vi "Sub_get_eigensol_and_sort_native_LABView.vi"(0 "Mass":T1, 1 "Stiffness":T1) -> (14 "Unsorted Eigenvalues":dbl[](array[numeric]), 15 "Sorted Eigenvalues":dbl[](array[numeric]), 16 "Unsorted Eigenvector Matrix":T1, 17 "Sorted Eigenvector Matrix":T1, 18 "Natural frequency":dbl[](array[numeric]))   [LabVIEW 2021]
uses:
  <vilib>/Analysis/Matrix/Datatypes/RealMatrix.ctl
  <vilib>/Analysis/Matrix/Numeric/Conversions/Matrix To Array - RM.vi
  <vilib>/Analysis/Matrix/Numeric/Conversions/Array To Matrix - RA2.vi
  <vilib>/Analysis/Matrix/NI_Matrix.lvlib
panel:
  # "Inputs"
  # "Outputs"
  # "This is a wrapper for Sub_Python_cmd_eigh.vi that sorts the eigen values returns the values of intrerest, IF YOU REPLACE the sub_vi this VI will sort the eigenvectors by ascending order according to their corresponding eigenvalues ASUMMING that the eigenvalues are stored as a vector V[i] corresonds to each column in eigenvector matrix W[:,i ]. Not all eigensolvers sort their eigenvalues in a simple ascending or descending order, or any order for that matter. This VI performs simple sort naive to any presupposed ordering.\n\n              - Alexander Vereen AFRL Summer scholars 2022"
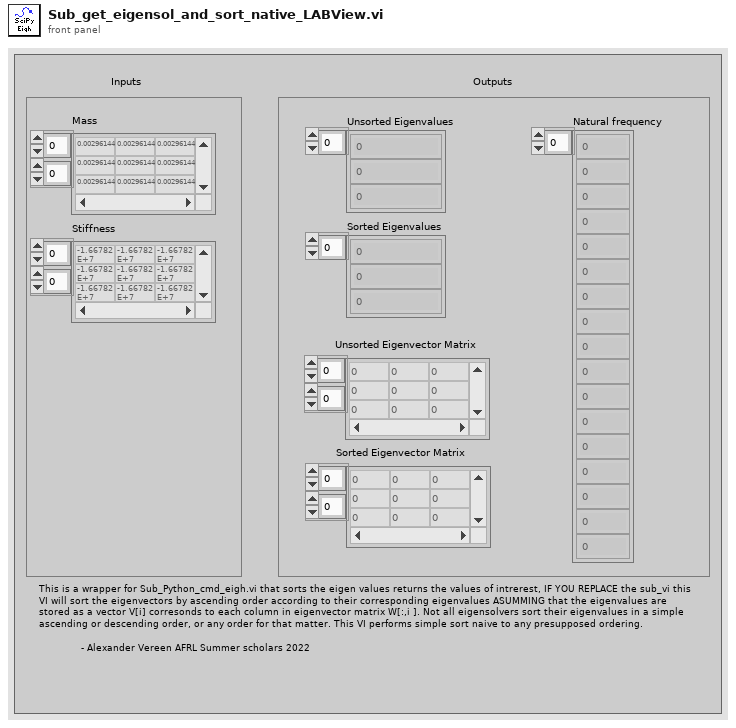
[diagram p1: front panel]
types:
  T1 = typedef "NI_Matrix.lvlib/RealMatrix.ctl" = dbl[][]
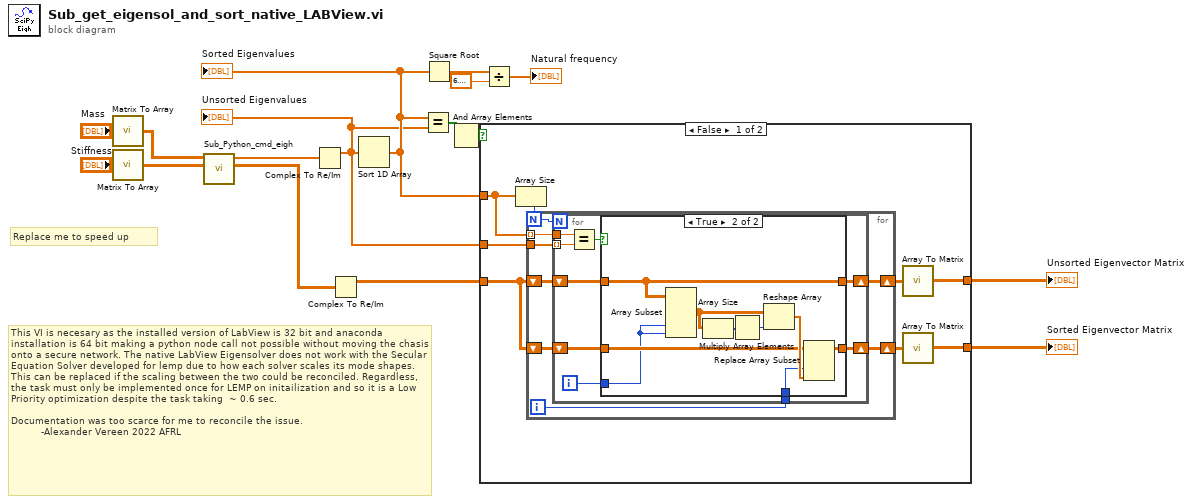
[diagram p0: block diagram]
diagram:
  # "Replace me to speed up"
  # "This VI is necesary as the installed version of LabView is 32 bit and anaconda installation is 64 bit making a python node call not possible without moving the chasis onto a secure network. The native LabView Eigensolver does not work with the Secular Equation Solver developed for lemp due to how each solver scales its mode shapes.  This can be replaced if the scaling between the two could be reconciled. Regardless, the task must only be implemented once for LEMP on initailization and so it is a Low Priority optimization despite the task taking  ~ 0.6 sec. \n\nDocumentation was too scarce for me to reconcile the issue.\n          -Alexander Vereen 2022 AFRL"
  n1 = call-poly <vilib>:"Matrix To Array.vi"("Real Matrix"="Mass") -> ("Real 2D Array"=w5:dbl[][])
  n2 = call-poly <vilib>:"Matrix To Array.vi"("Real Matrix"="Stiffness") -> ("Real 2D Array"=w6:dbl[][])
  n3 = call "Sub_Python_cmd_eigh.vi"("Stiff"=w6, "Mass"=w5) -> ("Eigenvectors"=w8:dbl[][], "Eigenvalues"=w9:dbl[])  [unwired: 8 in]
  n4 = Complex To Re/Im ("Complex To Cartesian.vi")(x + iy=w9) -> (x=w3:dbl[])  [unwired: 1 out]
  "Unsorted Eigenvalues" <- w3
  n5 = Complex To Re/Im ("Complex To Cartesian.vi")(x + iy=w8) -> (x=w12:dbl[][])  [unwired: 1 out]
  n6 = Sort 1D Array(array=w3) -> (sorted array=w4:dbl[])
  "Sorted Eigenvalues" <- w4
  n7 = Equal?(x=w4, y=w3) -> (x = y?=w2:bool[])
  n8 = Square Root ("Square Root.vi")(x=w4) -> (sqrt(x)=w16:dbl[])
  n9 = And Array Elements(Boolean array=w2) -> (logical AND=w1:bool)
  n10 = case shown="False" w1 {
    tunnel: [w21 w53] -> w14
    tunnel: [w20 w53] -> w13
    tunnel: w12 -> [w19 w53]
    tunnel: w3 -> [w18 _]
    tunnel: w4 -> [w17 _]
    frame False {
      n11 = Array Size(array=w17) -> (size(s)=w24:i32)
      n12 = for {
        N: w24 -> [w25]
        tunnel: w17 -> [w31] mode=indexing
        tunnel: w18 -> [w32]
        shift-right: [w29] -> w23
        shift-left: w19 -> [w30]
        shift-right: [w27] -> w22
        shift-left: w19 -> [w26]
        i -> [w28]
        n13 = for {
          N: w25 -> [_]
          tunnel: w32 -> [w40] mode=indexing
          tunnel: w31 -> [w41]
          shift-right: [w37] -> w29
          shift-left: w30 -> [w38]
          tunnel: w28 -> [w36]
          shift-right: [w34] -> w27
          shift-left: w26 -> [w33]
          i -> [w35]
          n14 = Equal?(x=w41, y=w40) -> (x = y?=w39:bool)
          n15 = case shown="True" w39 {
            tunnel: w38 -> [w43 w47]
            tunnel: [w43 w47] -> w37
            tunnel: w36 -> [_ w46]
            tunnel: w35 -> [_ w45]
            tunnel: [w42 w49] -> w34
            tunnel: w33 -> [w42 w48]
            frame False {
            }
            frame True {
              n16 = Array Subset(array=w47, index (col)=w45, length (col)=w45) -> (w50:dbl[][])  [unwired: 2 in]
              n17 = Array Size(array=w50) -> (size(s)=w51:i32[])
              n18 = Multiply Array Elements(1:w51) -> (0:w44:i32)
              n19 = Reshape Array(w50, w44) -> (w52:dbl[])
              n20 = Replace Array Subset(array=w48, new element=w52, index (col)=w46) -> (w49:dbl[][])  [unwired: 1 in]
            }
          }
        }
      }
      n21 = call-poly <vilib>:"Array To Matrix.vi"("Real 2D Array"=w23) -> ("Real Matrix"=w20:T1)
      n22 = call-poly <vilib>:"Array To Matrix.vi"("Real 2D Array"=w22) -> ("Real Matrix"=w21:T1)
    }
    frame True {
    }
  }
  "Unsorted Eigenvector Matrix" <- w13
  "Sorted Eigenvector Matrix" <- w14
  n23 = Divide(x=w16, y=6.283185307179586) -> (x/y=→"Natural frequency":dbl[])
